vi "ElectrodeInquireStatus.vi"(8 "error in (no error)":errorcluster, 11 "Electrode in":refnum<class "Electrode.lvclass">) -> (0 "error out":errorcluster, 2 "Electrode Activated?":bool=TRUE, 3 "Electrode out":refnum<class "Electrode.lvclass">)   [LabVIEW 2012, in "Electrode.lvclass"]
uses:
  Electrode.lvclass
  Electrode.lvclass/Electrode.ctl
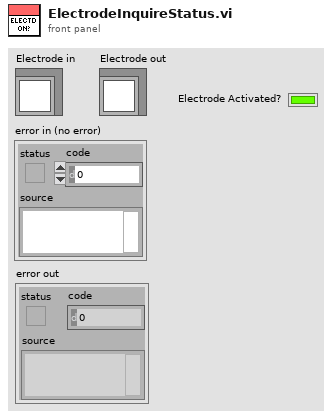
[diagram p1: front panel]
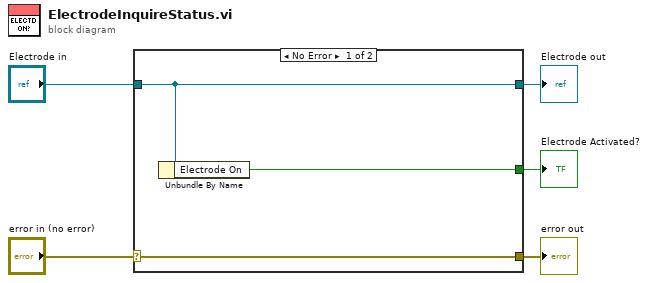
[diagram p0: block diagram]
diagram:
  n1 = case shown="No Error" "error in (no error)" {
    selector: "error in (no error)" -> [w8 w9]
    tunnel: [w8 w9] -> w4
    tunnel: [w7 w10] -> w2
    tunnel: "Electrode in" -> [w7 w10]
    tunnel: [w6 _] -> w1
    frame No Error {
      n2 = Unbundle By Name(w7) -> ("Electrode On"=w6:bool)
    }
    frame Error {
    }
  }
  "error out" <- w4
  "Electrode out" <- w2
  "Electrode Activated?" <- w1
